vi "ListNamedPositions.vi"(8 "error in (no error)":errorcluster, 11 "XYStage":refnum<class "XYStage.lvclass">) -> (0 "error out":errorcluster, 1 "Positions":T1[](array[typedef]), 2 "Names":string[](array[string]), 3 "XYStage out":refnum<class "XYStage.lvclass">)   [LabVIEW 2013, in "XYStage.lvclass"]
doc: "---------------------------------------------------------------\nJKI State Machine Objects™\nhttp://jki.net/state-machine-objects/\nCopyright (C) 2005-2015, JKI <info@jki.net>\nALL RIGHTS RESERVEDJKI State Machine Objects (SMO) 1.0.0.4\nJKI - JKI\nCopyright (c) 2015, JKI"
uses:
  XYStage.lvclass
  <vilib>/JKI/JKI SMO/SMO.Dictionary/SMO.Dictionary.lvclass
  Typedefs/(real)Coords--Cluster.ctl
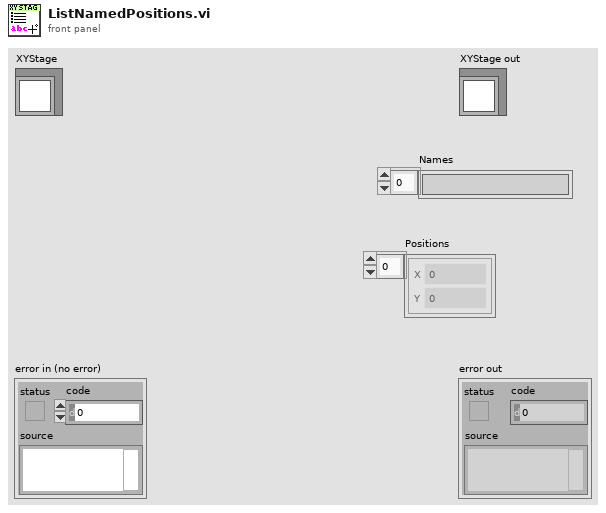
[diagram p1: front panel]
types:
  T1 = typedef "XYStage.lvclass/(real)Coords--Cluster.ctl" = cluster{"X":dbl, "Y":dbl}
  T2 = typedef "XYStage.lvclass/Dependencies--Cluster.ctl" = cluster{"Positions":refnum<class "SMO.Dictionary.Variant.lvclass">}
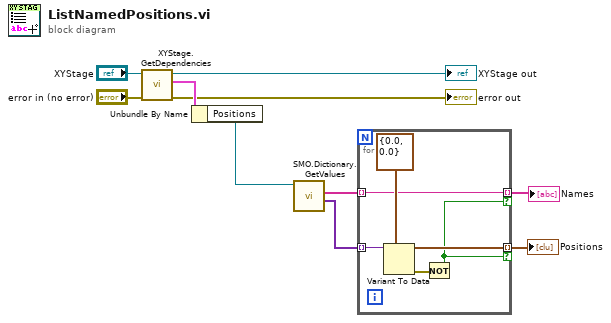
[diagram p0: block diagram]
diagram:
  n1 = call "XYStage.GetDependencies.vi"("error in (no error)"="error in (no error)", "XYStage"="XYStage") -> ("error out"=→"error out":errorcluster, "Dependencies"=w10:T2, "XYStage out"=→"XYStage out":refnum<class "XYStage.lvclass">)  [unwired: 7 in]
  n2 = Unbundle By Name(w10) -> ("Positions"=w5:refnum<class "SMO.Dictionary.Variant.lvclass">)
  n3 = call <vilib>:"SMO.Dictionary.GetValues.vi"("SMO.Dictionary"=w5) -> ("Values"=w4:variant[], "Keys out"=w2:string[])  [unwired: 6 in, 3 out]
  n4 = for {
    tunnel: w4 -> [w15] mode=indexing
    tunnel: [w14] -> w3 mode=indexing if=w11
    tunnel: w2 -> [w12] mode=indexing
    tunnel: [w12] -> w1 mode=indexing if=w11
    n5 = Variant To Data(type=T1 {"X"=0.0, "Y"=0.0} ("Coords"), Variant=w15) -> (data=w14:T1, error out=w16:errorcluster)  [unwired: 1 in]
    n6 = Not(x=w16) -> (.not. x?=w11:bool)
  }
  "Names" <- w1
  "Positions" <- w3
